vi "ReadConcTempPressureVer08.vi"() -> ()   [LabVIEW 2011]
uses:
  <vilib>/Utility/error.llb/DialogType.ctl
  <vilib>/Analysis/NI_AALBase.lvlib
panel:
  out "CPCconc":dbl=5620.0
  out "Smps Setting String":string
  in  "Allow SMPS scan":bool
  out "Saving in Progress":i32(slide) caption="Saving" scale=0.0..9.0
  out "Pressure (Hectopascal)":dbl=1011.5068458586213 format="%#.2f"
  out "Number Samples of Press.":dbl format="%.1f"
  out "Std error Press. to file (hpas)":dbl format="%.2f"
  out "Mean Press. to file (hpas)":dbl format="%.2f"
  in  "Std Press. error tolerance(%)":dbl=0.1 format="%.1f"
  out "Mean Pressure":dbl format="%.1f"
  out "Std Error Pressure (%)":dbl format="%.2f"
  out "Pressure Graph":cluster{"mean":dbl, dbl}(graph)={"mean"=1011.5068458586213, 1011.5068458586213} caption="Waveform Chart"
  out "Temperature(Celcius)":dbl=22.3189775953034 format="%#.2f"
  out "Number Samples of Temp":dbl format="%.1f"
  out "Std error Temp to file (deg)":dbl format="%.1f"
  out "Mean Temp to file (deg)":dbl format="%#.0f"
  in  "Std Temp error tolerance(%)":dbl=0.1 format="%.1f"
  out "Mean Temperature":dbl format="%.2f"
  out "Std Error Temp (%)":dbl format="%.2f"
  out "Temperature Graph":cluster{"mean":dbl, dbl}(graph)={"mean"=22.3189775953034, 22.3189775953034} caption="Waveform Chart"
  in  "CPC port":refnum<visa-resource-name>="COM4"
  out "Conc. (N/cm^3)":dbl=5620.0 format="%.1f"
  out "Number Samples of Conc.":dbl format="%.1f"
  out "Std error to file (N/cm^3)":dbl format="%.1f"
  out "Mean conc. to file (N/cm^3)":dbl format="%.2f"
  out "output array 2":dbl[](array[numeric])
  out "output 2":dbl
  out "output 1":dbl
  out "Std Error Concentration":dbl format="%.1f"
  in  "Std Conc. error tolerance(%)":dbl=0.1 format="%.1f"
  out "Std Concentration":dbl format="%.1f"
  out "Mean Conc.":dbl format="%.1f"
  out "Std Error Conc. (%)":dbl format="%.2f"
  out "output array":dbl[](array[numeric])=[5620.0, 5680.0, 5660.0, 5740.0, nan, 0.0, 0.0, 0.0, 0.0, 0.0, 0.0, 0.0, 0.0, 0.0, 0.0, 0.0, 0.0, 0.0, 0.0, 0.0, 0.0, 0.0, 0.0, 0.0, 0.0, 0.0, 0.0, 0.0, 0.0, 0.0]
  in  "Running Average Time(sec)":i32=30
  out "Particle Concentration from CPC":cluster{"mean":dbl, dbl}(graph)={"mean"=5620.0, 5620.0} caption="Waveform Chart"
  in  "OK":bool
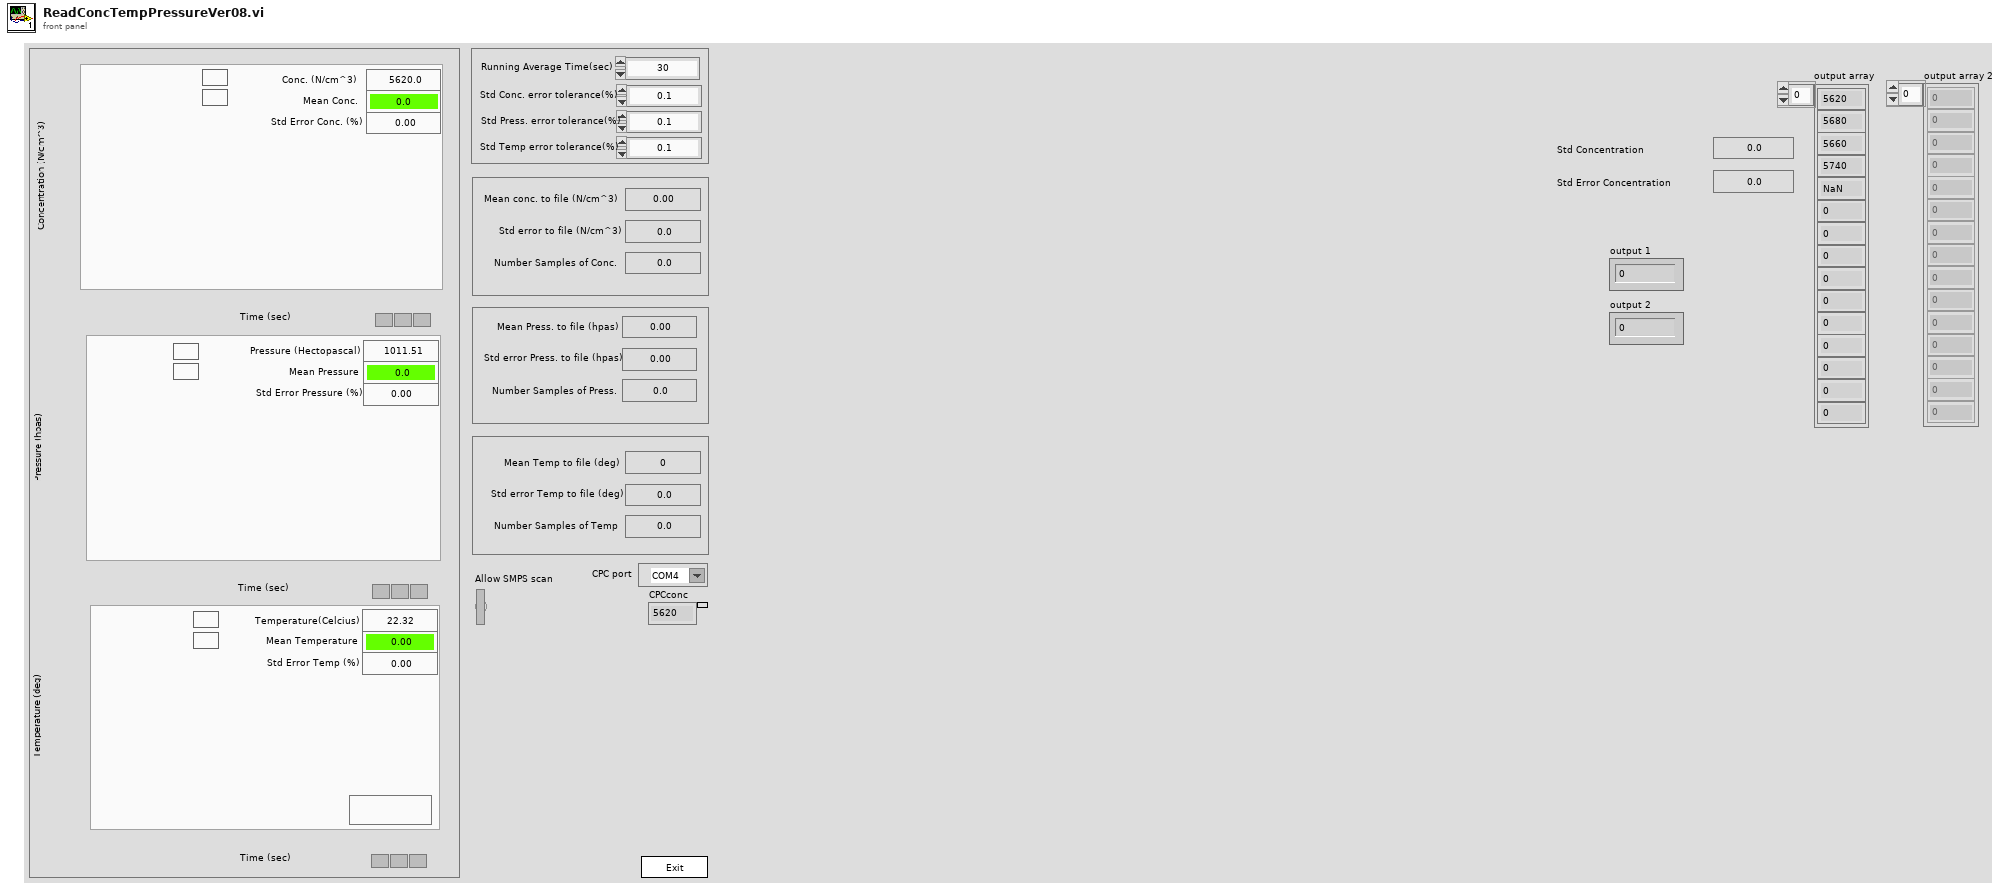
[diagram p1: front panel]
types:
  T1 = enum32{"invalid app kind", "Development System", "Run Time System", "Student Edition", "Embedded LabVIEW", "Evaluation", "Custom"}
  T2 = enum32{"Invalid", "Standard", "Closed", "Hidden", "Minimized", "Maximized"}
  T3 = cluster{"Core":cluster{"Current VI Reference":refnum<vi>, "Close Panel on Exit?":bool}, dbl[], "Running Average Time(sec)":i32, dbl[], "element":dbl, "dimension size":i32, "input file":path, "input file":path, "dup CPC port":refnum<visa-resource-name>, "CPC model":string, "input file":path, "input file":path, cluster{dbl[], dbl[], "element":dbl}, cluster{dbl[], dbl[], "element":dbl}}
  T4 = typedef "DialogType.ctl" = u16
  T5 = cluster{"Current VI Reference":refnum<vi>, "Close Panel on Exit?":bool}
  T6 = cluster{"concentration part/cm3":dbl, "concentration part/cm3":dbl}
  T7 = cluster{"concentration part/cm3":dbl, "mean":dbl}
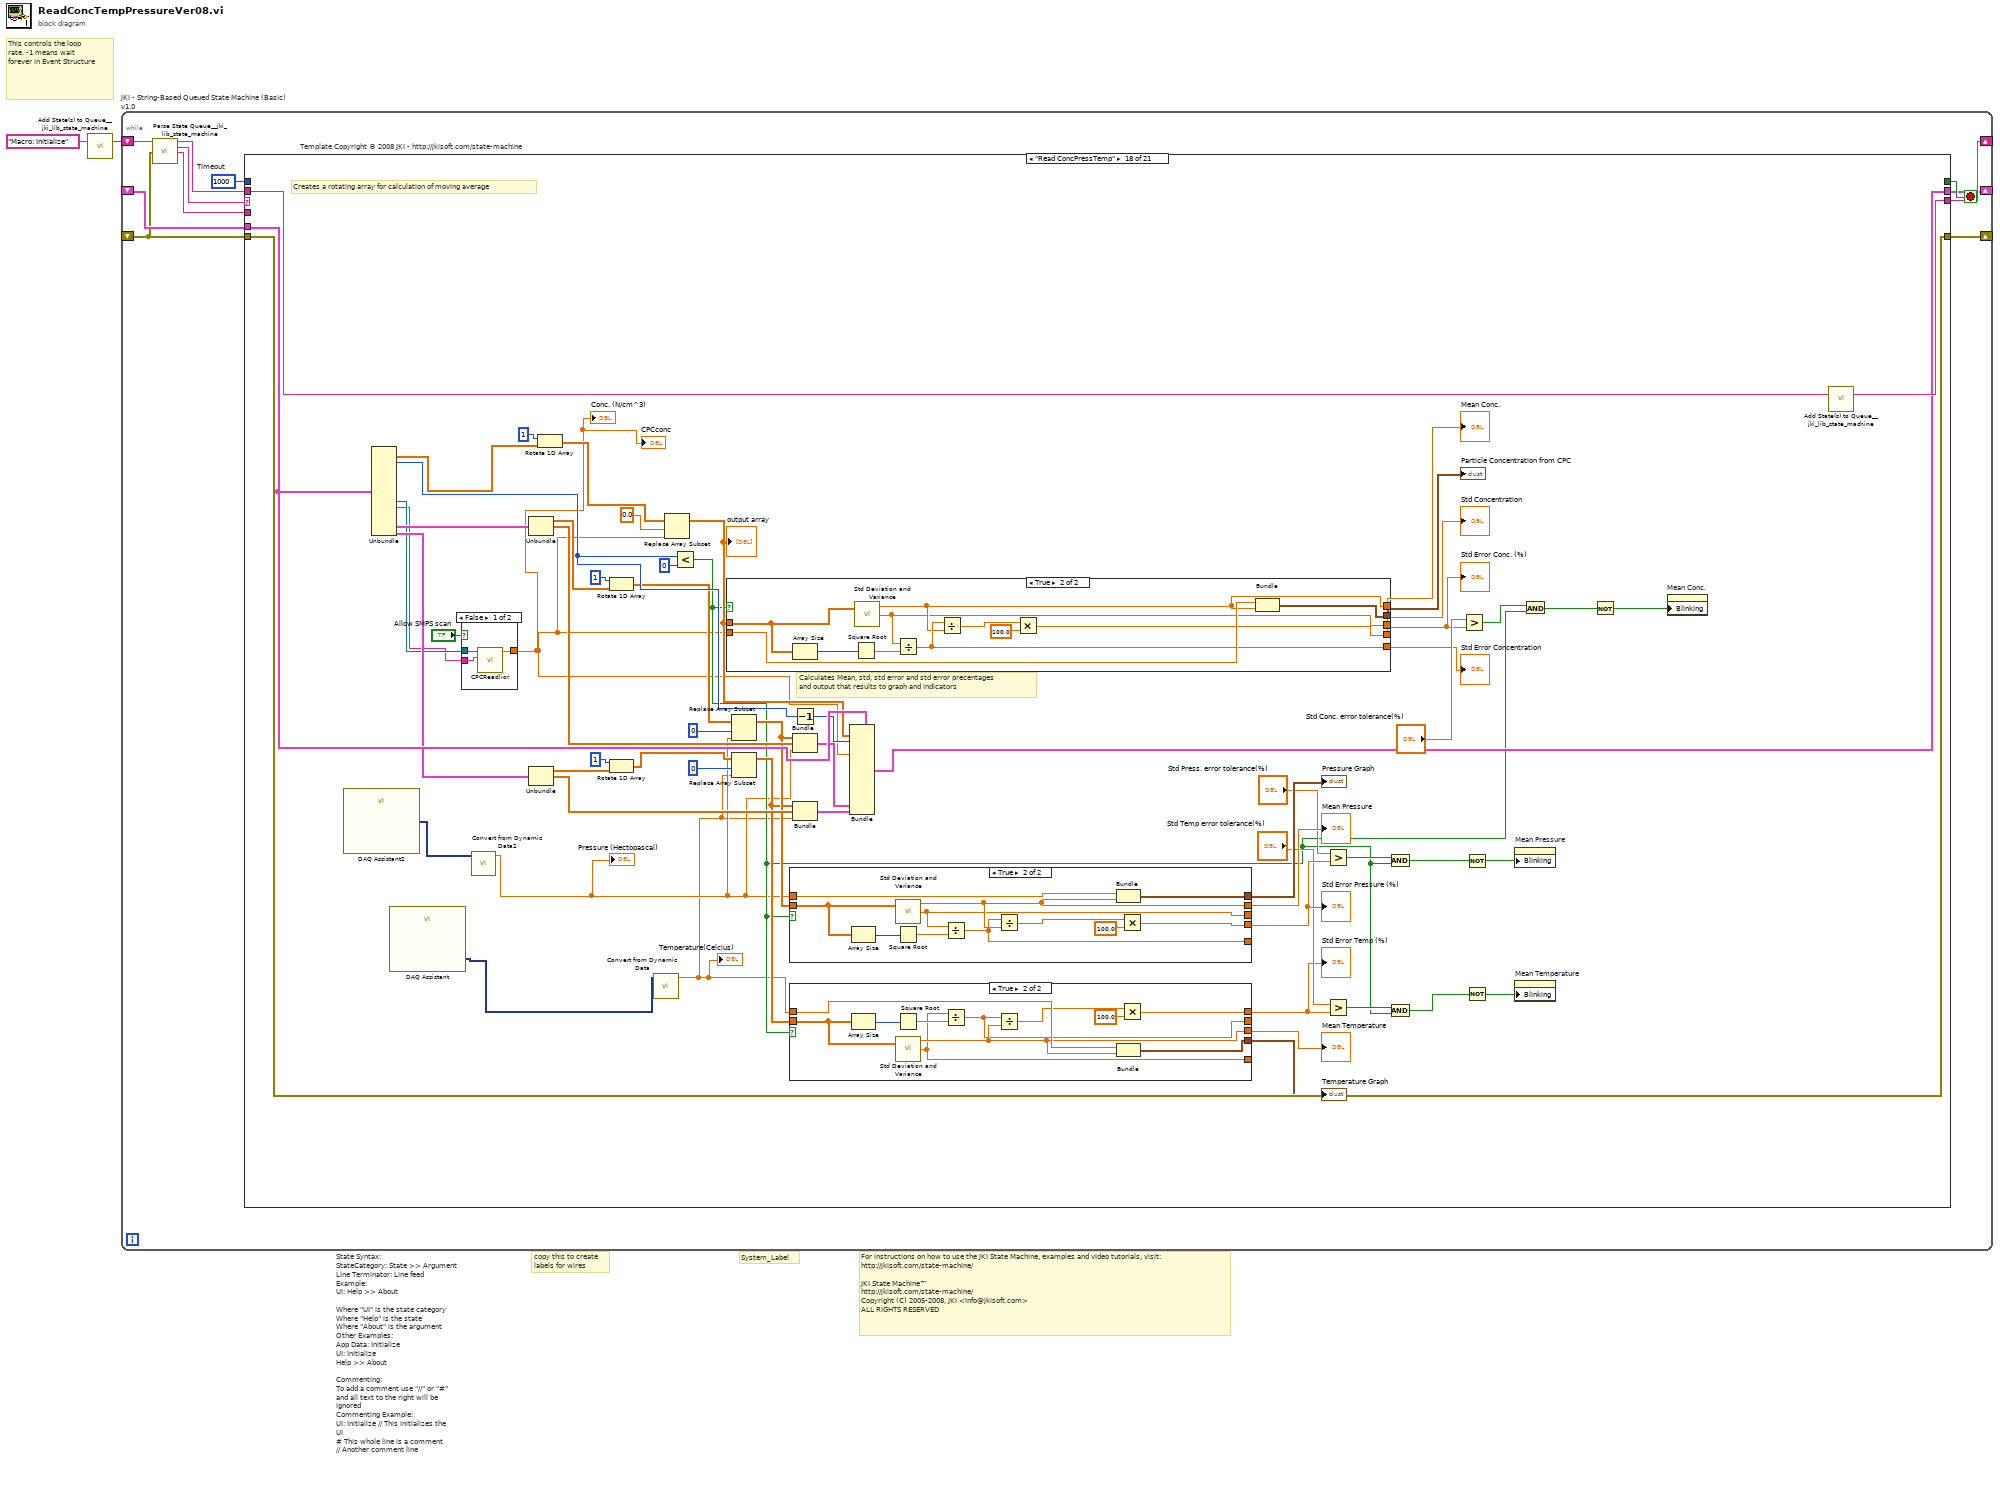
[diagram p0: block diagram]
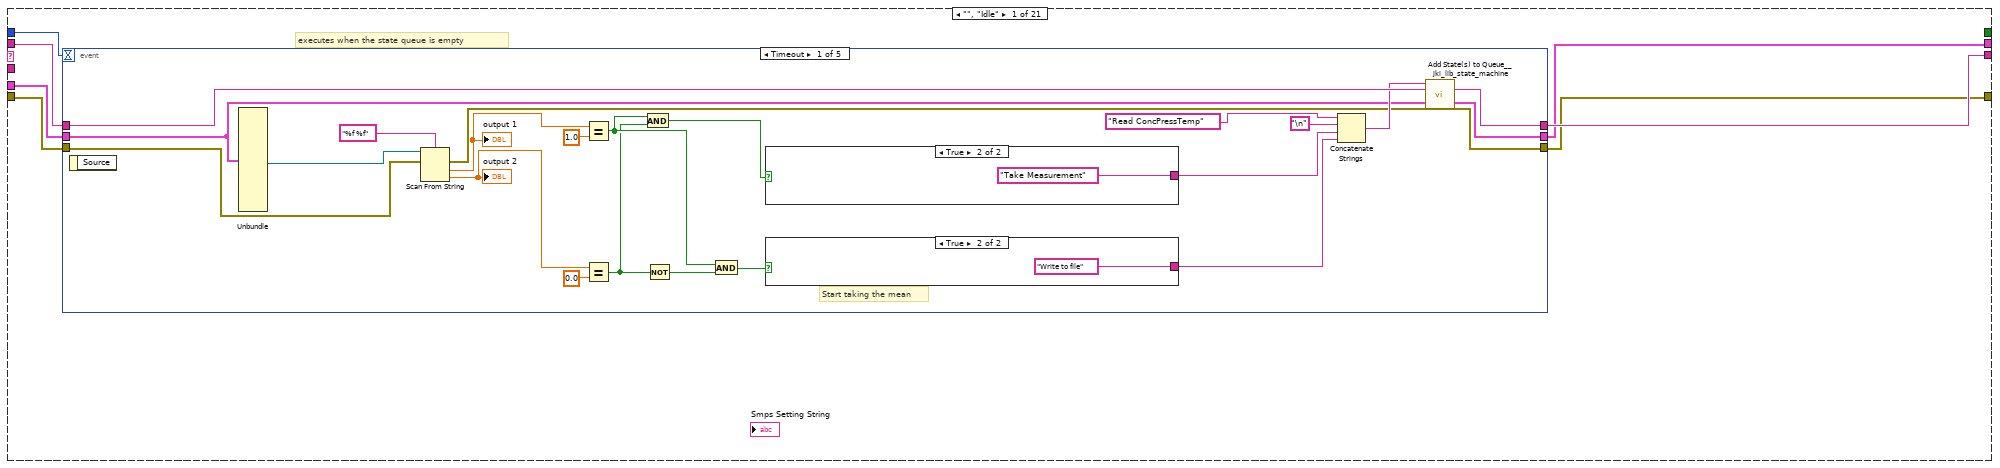
[diagram p2: hidden frame]
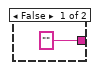
[diagram p3: hidden frame]
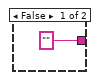
[diagram p4: hidden frame]
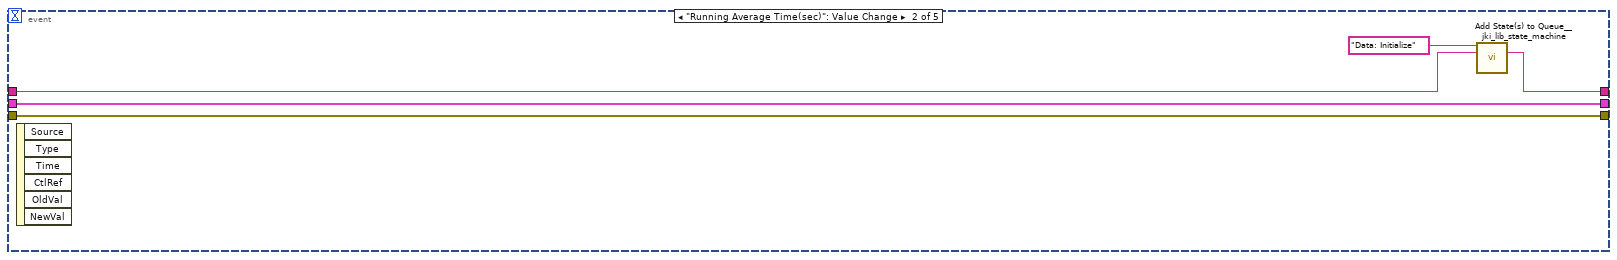
[diagram p5: hidden frame]
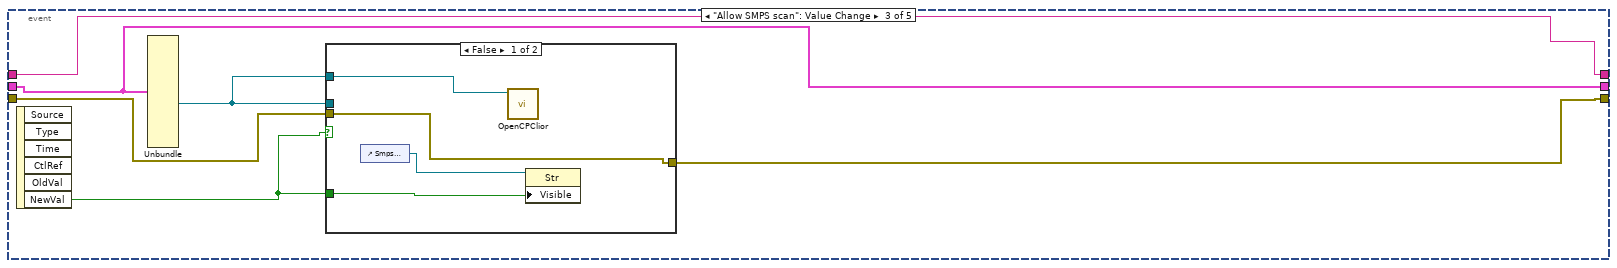
[diagram p6: hidden frame]
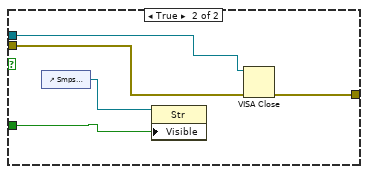
[diagram p7: hidden frame]
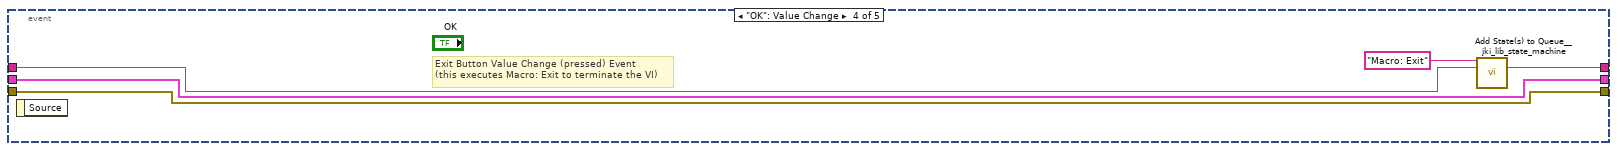
[diagram p8: hidden frame]
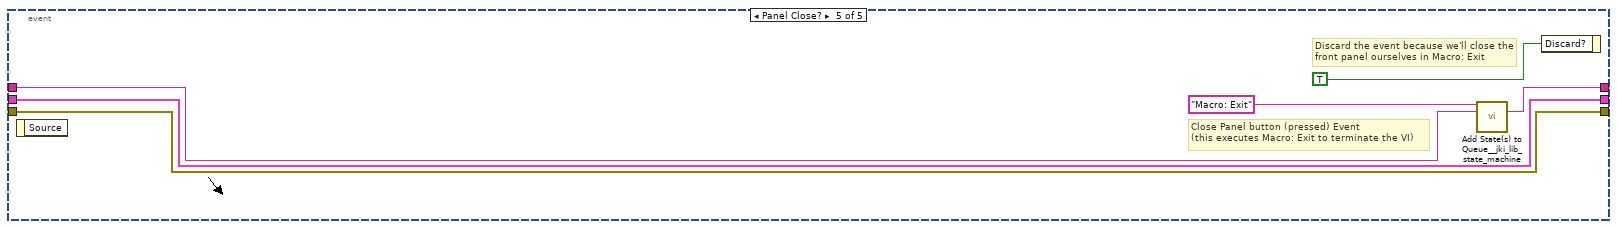
[diagram p9: hidden frame]
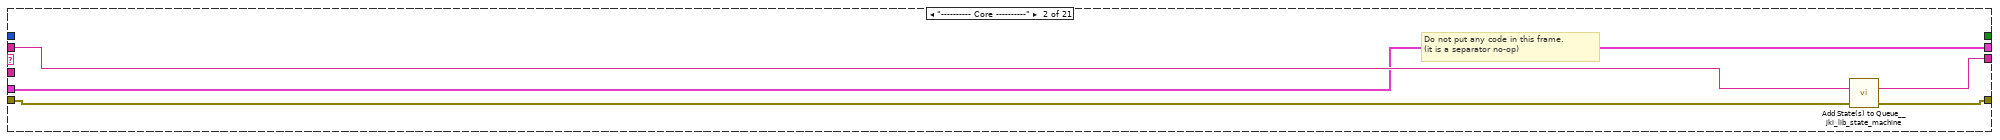
[diagram p10: hidden frame]
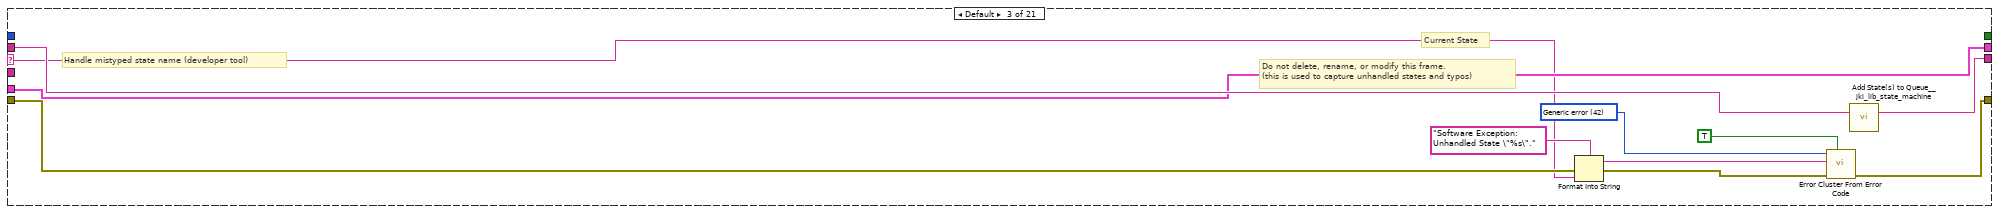
[diagram p11: hidden frame]
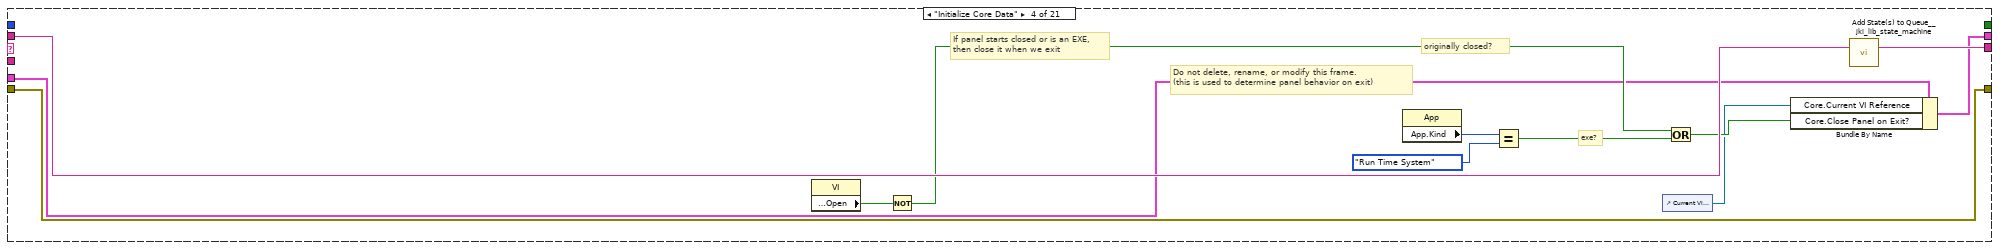
[diagram p12: hidden frame]
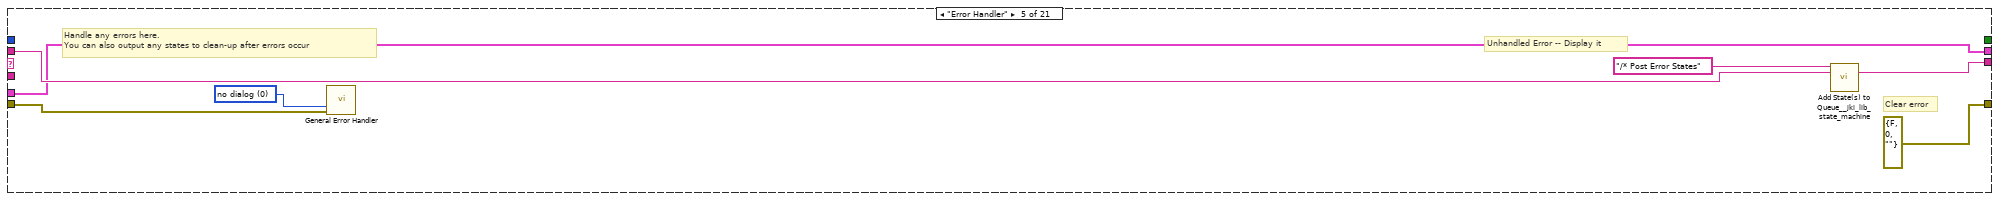
[diagram p13: hidden frame]
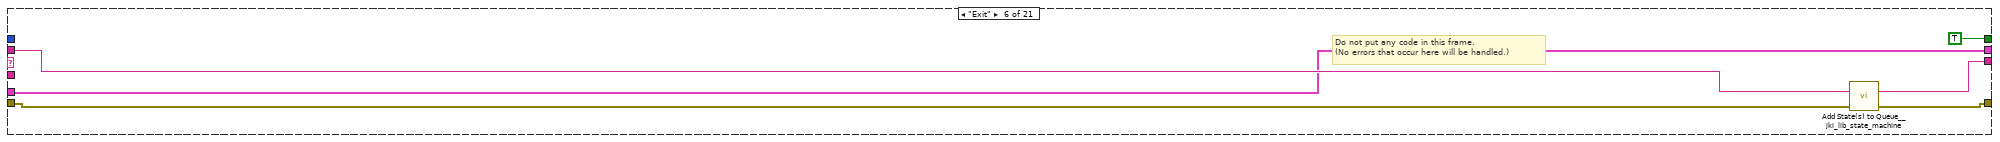
[diagram p14: hidden frame]
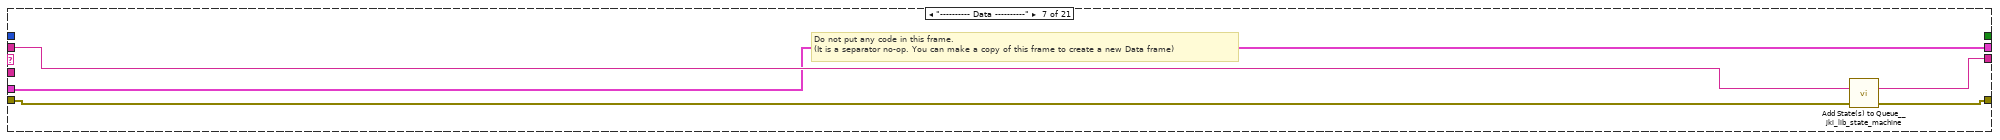
[diagram p15: hidden frame]
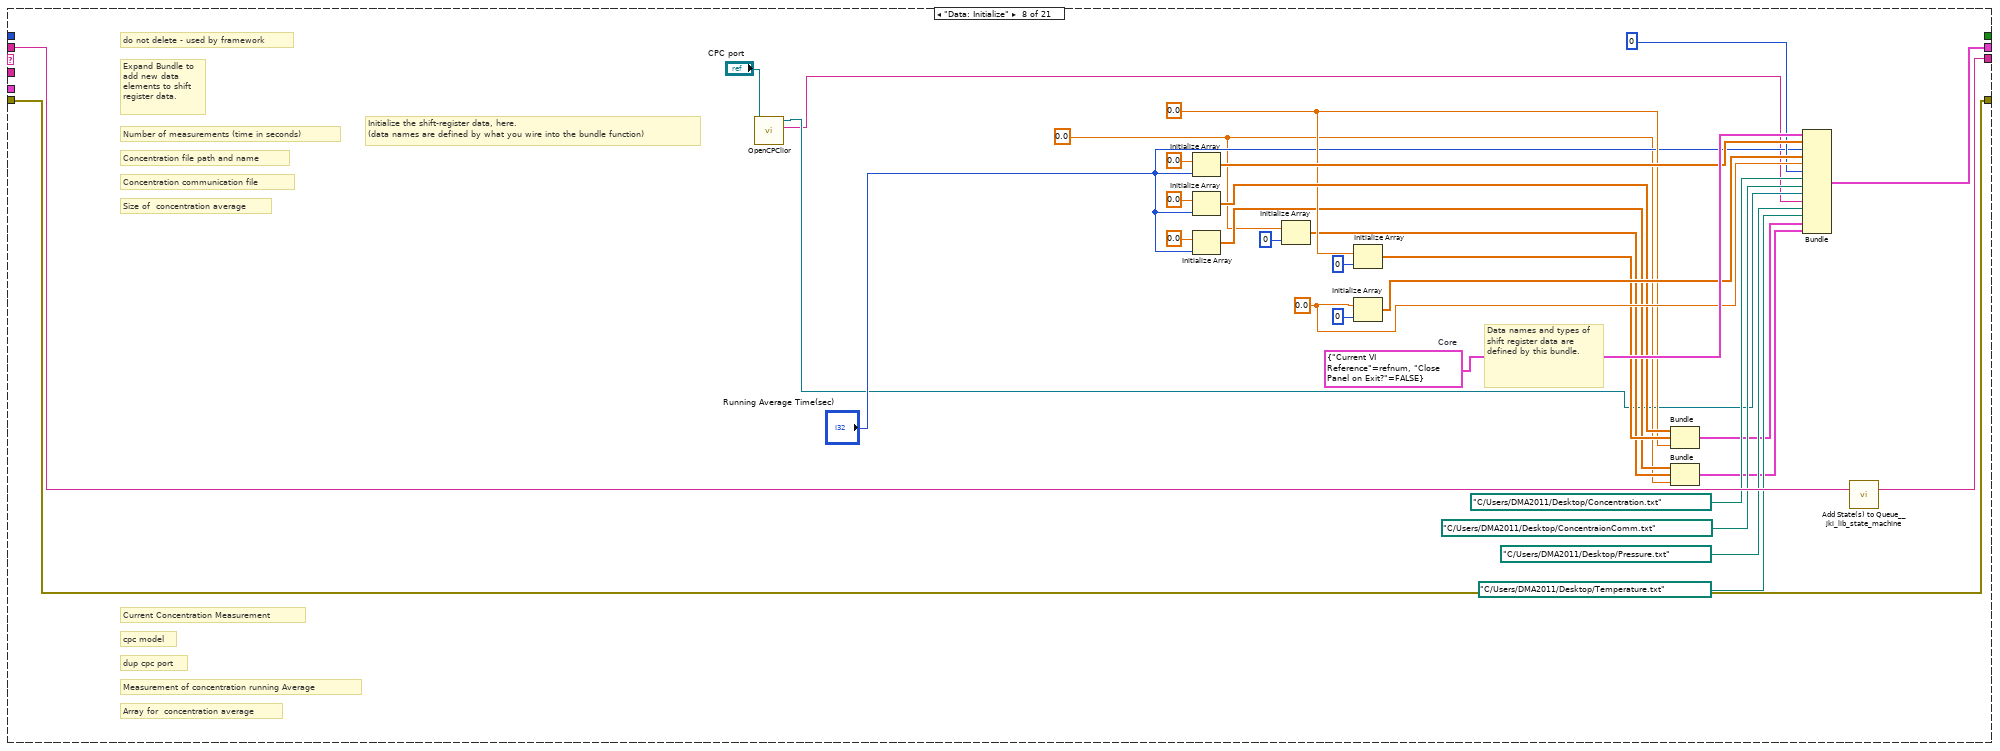
[diagram p16: hidden frame]
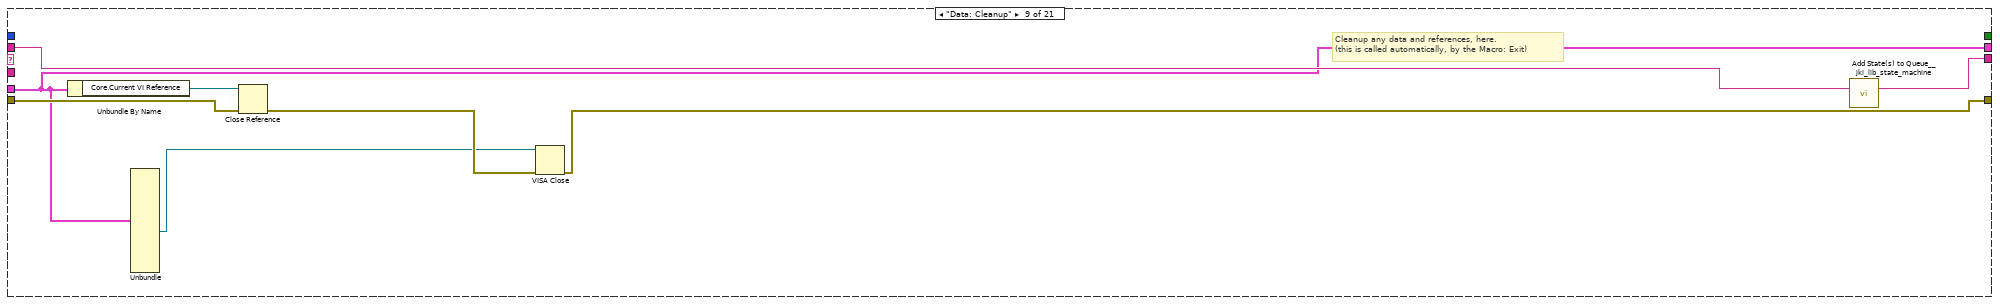
[diagram p17: hidden frame]
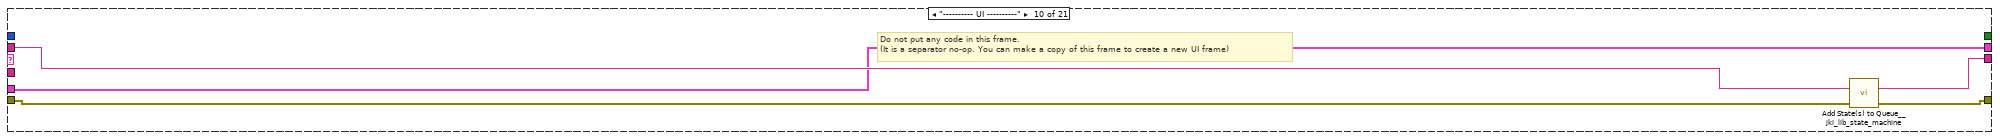
[diagram p18: hidden frame]
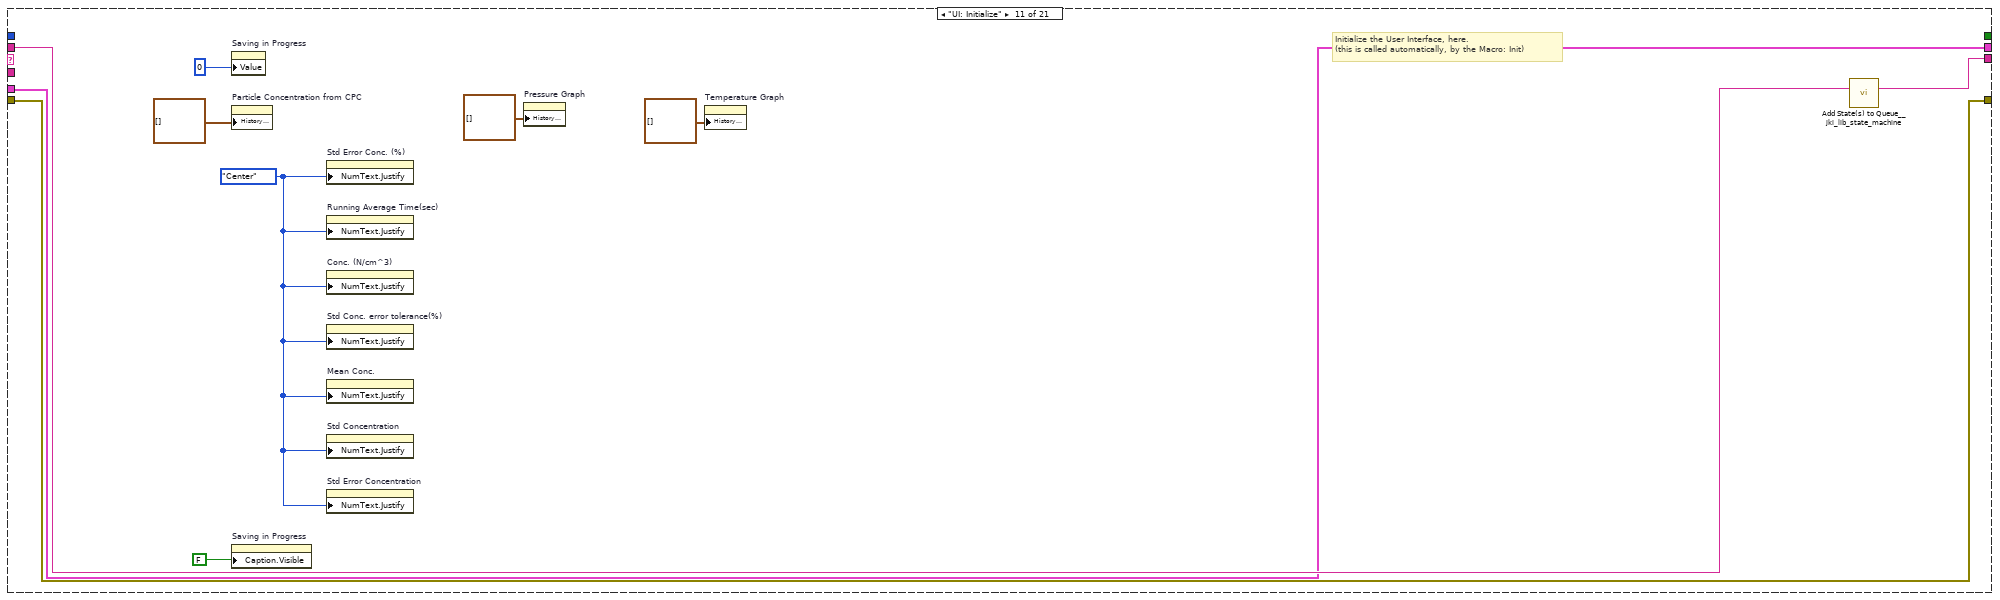
[diagram p19: hidden frame]
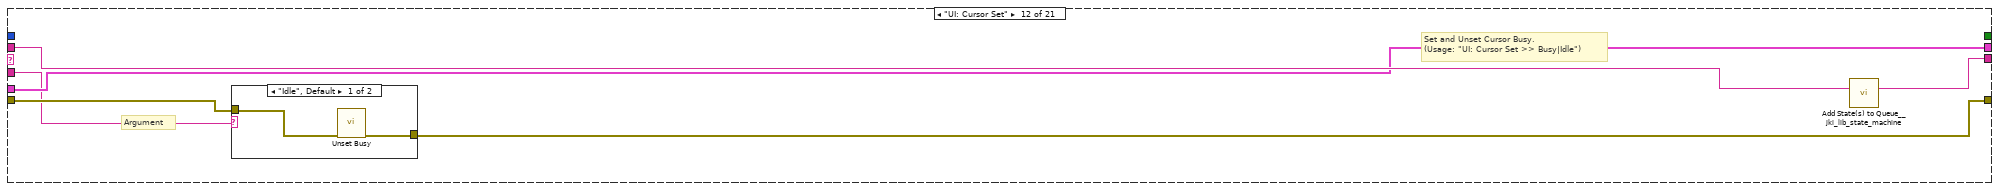
[diagram p20: hidden frame]
diagram:
  # "For instructions on how to use the JKI State Machine, examples and video tutorials, visit:\nhttp://jkisoft.com/state-machine/\n\nJKI State Machine™\nhttp://jkisoft.com/state-machine/\nCopyright (C) 2005-2008, JKI <info@jkisoft.com>\nALL RIGHTS RESERVED"
  # "State Syntax:\nStateCategory: State >> Argument\nLine Terminator: Line feed\nExample:\nUI: Help >> About\n\nWhere \"UI\" is the state category\nWhere \"Help\" is the state\nWhere \"About\" is the argument\nOther Examples:\nApp Data: Initialize\nUI: Initialize\nHelp >> About\n\nCommenting:\nTo add a comment use \"//\" or \"#\" and all text to the right will be ignored\nCommenting Example:\nUI: Initialize // This initializes the UI\n# This whole line is a comment\n// Another comment line"
  # "copy this to create labels for wires"
  # "This controls the loop rate. -1 means wait forever in Event Structure"
  # "System_Label"
  n1 = call <vilib>:"Add State(s) to Queue__jki_lib_state_machine.vi"("State(s) in (\"\")"="Macro: Initialize") -> ("States Out"=w2:string)  [unwired: 14 in]
  n2 = while "JKI - String-Based Queued State Machine (Basic) v1.0" {
    shift-right: [w6] -> _
    shift-left: _ -> [w5]
    shift-right: [w9] -> _
    shift-left: _ -> [w3]
    shift-right: [w8] -> _
    shift-left: w2 -> [w10]
    stop <- w7 stop-if-true
    w4 = 1000  # Timeout
    # "Template Copyright © 2008 JKI - http://jkisoft.com/state-machine"
    n3 = call <vilib>:"Parse State Queue__jki_lib_state_machine.vi"("State Queue"=w10, "Error In (no error)"=w3) -> ("Remaining States"=w12:string, "Current State"=w13:string, "Arguments"=w11:string)  [unwired: 11 in]
    n4 = case shown="\"Read ConcPressTemp\"" w13 {
      selector: w13 -> [_ _ w81 _ _ _ _ _ _ _ _ _ _ _ _ _ _ _ _ _ _]
      tunnel: w12 -> [w20 w80 w85 w103 w110 w115 w119 w150 w158 w162 w172 w178 w189 w215 w220 w230 w234 w295 w345 w375 w435]
      tunnel: w11 -> [_ _ _ _ _ _ _ _ _ _ _ w173 w183 _ _ _ _ _ _ _ _]
      tunnel: w5 -> [w18 w77 w83 w94 w107 w113 w116 _ w152 w159 w170 w176 w185 w212 w217 w227 w231 w291 w342 w369 w424]
      tunnel: [w17 w78 w87 w100 errorcluster {"status"=FALSE, "code"=0, "source"=""} ("error out") w112 w117 w147 w153 w160 w169 w174 w186 w213 w218 w228 w232 w293 w343 w373 w398] -> w9
      tunnel: w3 -> [w16 w78 w86 w100 w106 w112 w117 w147 w155 w160 w169 w175 w187 w213 w218 w228 w232 w293 w343 w373 w413]
      tunnel: [w19 w79 w84 w102 w109 w114 w118 w149 w157 w161 w171 w177 w188 w214 w219 w229 w233 w294 w344 w374 w434] -> w8
      tunnel: [_ _ _ _ _ TRUE _ _ _ _ _ _ _ _ _ _ _ _ _ _ _] -> w7
      tunnel: [w15 w77 w83 w101 w107 w113 w116 w148 w152 w159 w170 w176 w185 w212 w217 w227 w231 w292 w342 w368 w423] -> w6
      tunnel: w4 -> [w14 _ _ _ _ _ _ _ _ _ _ _ _ _ _ _ _ _ _ _ _]
      frame "", "Idle" {
        # "executes when the state queue is empty"
        n5 = event shown="[0] Timeout" {
          selector: _ -> [_ _ _ _ _]
          dyn-events: _ -> [_ _ _ _ _]
          timeout: w14 -> [_ _ _ _ _]
          tunnel: w20 -> [w41 w50 w53 w70 w76]
          tunnel: [w40 w49 w53 w69 w75] -> w19
          tunnel: w18 -> [w24 w47 w52 w67 w73]
          tunnel: [w21 w48 w55 w68 w74] -> w17
          tunnel: w16 -> [w22 w48 w56 w68 w74]
          tunnel: [w24 w47 w52 w67 w73] -> w15
          event Timeout {
            # "Start taking the mean"
            n6 = event-data() -> ()  [unwired: 1 in, 1 out]
            n7 = Unbundle(w24) -> ("input file"=w23:path)  [unwired: 13 out]
            n8 = Scan From String("%f %f" ("format string"), w23, w22) -> (w21:errorcluster, output 1=w38:dbl, output 2=w35:dbl)  [unwired: 2 in, 1 out]
            "output 1" <- w38
            "output 2" <- w35
            n9 = Equal?(x=w38, y=1.0) -> (x = y?=w29:bool)
            n10 = Equal?(x=w35, y=0.0) -> (x = y?=w27:bool)
            n11 = And(x=w29, y=w27) -> (x .and. y?=w34:bool)
            n12 = Not(x=w27) -> (.not. x?=w28:bool)
            n13 = And(x=w29, y=w28) -> (x .and. y?=w26:bool)
            n14 = case shown="True" w34 {
              tunnel: ["" ("State(s) in Front (\"\")") "Take Measurement" ("State(s) in Front (\"\")")] -> w30
              frame False {
              }
              frame True {
              }
            }
            n15 = case shown="True" w26 {
              tunnel: ["" ("State(s) in Front (\"\")") "Write to file" ("State(s) in Front (\"\")")] -> w25
              frame False {
              }
              frame True {
              }
            }
            n16 = Concatenate Strings("Read ConcPressTemp" ("State(s) in Front (\"\")"), "\n", w30, w25) -> (w33:string)
            n17 = call <vilib>:"Add State(s) to Queue__jki_lib_state_machine.vi"("State(s) in Front (\"\")"=w33, "State(s) in (\"\")"=w41) -> ("States Out"=w40:string)  [unwired: 13 in]
          }
          event "Running Average Time(sec)": Value Change {
            n18 = event-data() -> ()  [unwired: 1 in, 6 out]
            n19 = call <vilib>:"Add State(s) to Queue__jki_lib_state_machine.vi"("State(s) in Front (\"\")"="Data: Initialize" ("State(s) in Front (\"\")"), "State(s) in (\"\")"=w50) -> ("States Out"=w49:string)  [unwired: 13 in]
          }
          event "Allow SMPS scan": Value Change {
            n20 = event-data() -> ("NewVal"=w51:bool)  [unwired: 1 in, 5 out]
            n21 = Unbundle(w52) -> ("dup CPC port"=w54:refnum<visa-resource-name>)  [unwired: 13 out]
            n22 = case shown="False" w51 {
              tunnel: w54 -> [_ w65]
              tunnel: w56 -> [w59 w64]
              tunnel: [w59 w63] -> w55
              tunnel: w54 -> [w60 _]
              tunnel: w51 -> [w57 w61]
              frame False {
                n23 = control-ref of="Smps Setting String"() -> (w58:refnum<vi>)
                n24 = call "OpenCPClior.vi"("CPC port"=w60) -> ()  [unwired: 8 in, 3 out]
                n25 = property on="Property Node" class="Str"(reference=w58, "Visible"=w57) -> ()  [unwired: 1 in, 2 out]
              }
              frame True {
                n26 = control-ref of="Smps Setting String"() -> (w62:refnum<vi>)
                n27 = property on="Property Node" class="Str"(reference=w62, "Visible"=w61) -> ()  [unwired: 1 in, 2 out]
                n28 = VISA Close(VISA resource name=w65, error in (no error)=w64) -> (error out=w63:errorcluster)
              }
            }
          }
          event "OK": Value Change {
            # "Exit Button Value Change (pressed) Event\n(this executes Macro: Exit to terminate the VI)"
            n29 = event-data() -> ()  [unwired: 1 in, 1 out]
            n30 = call <vilib>:"Add State(s) to Queue__jki_lib_state_machine.vi"("State(s) in Front (\"\")"="Macro: Exit", "State(s) in (\"\")"=w70) -> ("States Out"=w69:string)  [unwired: 13 in]
          }
          event Panel Close? {
            # "Discard the event because we'll close the front panel ourselves in Macro: Exit"
            # "Close Panel button (pressed) Event\n(this executes Macro: Exit to terminate the VI)"
            n31 = event-data() -> ()  [unwired: 1 in, 1 out]
            n32 = call <vilib>:"Add State(s) to Queue__jki_lib_state_machine.vi"("State(s) in Front (\"\")"="Macro: Exit", "State(s) in (\"\")"=w76) -> ("States Out"=w75:string)  [unwired: 13 in]
            n33 = event-data("Discard?"=TRUE) -> ()  [unwired: 1 in, 1 out]
          }
        }
      }
      frame "---------- Core ----------" {
        # "Do not put any code in this frame.\n(it is a separator no-op)"
        n34 = call <vilib>:"Add State(s) to Queue__jki_lib_state_machine.vi"("State(s) in (\"\")"=w80) -> ("States Out"=w79:string)  [unwired: 14 in]
      }
      frame Default {
        w90 = 42 items=["No error", "Argument error", "Memory is full", "Out of zone", "End of file", "File already open", "Generic file I/O error", "File not found", "File permission error", "Disk is full", "Duplicate path", "Too many files open", "System feature not enabled", "Resource file not found", "Cannot add resource", "Resource not found", "Image not found", "Image memory error", "Pen does not exist", "Config type invalid", "Config token not found", "Config parse error", "Config memory error", "Bad external code format", "Bad external code offset", "External code not present", "Null window", "Destroy window error", "Null menu", "Print aborted", "Bad print record", "Print driver error", "Windows error during printing", "Memory error during printing", "Print dialog error", "Generic print error", "Invalid device refnum", "Device not found", "Device parameter error", "Device unit error", "Cannot open device", "Device call aborted", "Generic error", "Cancelled by user", "Object ID too low", "Object ID too high", "Object not in heap", "Unknown heap", "Unknown object (invalid DefProc)", "Unknown object (DefProc not in table)", "Message out of range", "Invalid (null) method", "Unknown message", "Manager call not supported", "Bad address", "Network operation in progress", "Network operation timed out", "Connection is busy", "Network attribute not supported", "Network error", "Address in use", "System out of memory", "Connection aborted", "Connection refused", "Not connected", "Already connected", "Connection closed", "Initialization error (interapplication manager)", "Bad occurrence", "Wait on unbound occurrence handler", "Occurrence queue overflow", "Datalog type conflict", "Unused", "Unrecognized type (interapplication manager)", "Memory corrupt", "Failed to make temporary DLL", "Old CIN version", "Drag socket not found", "Failed to load drop-object", "Failed to register OLE object", "Failed to release OLE object", "Format specifier type mismatch", "Unknown format specifier", "Too few format specifiers", "Too many format specifiers", "Scan failed", "Newer CIN version", "Error converting to variant", "Runtime menu error", "Password tampered", "Variant attribute not found", "Incompatible variant data type", "Event data is not available", "Event Store is not present", "Occurrence is not found", "Event Queue is not created", "Event info is not available", "Refnum passed is NULL", "Error retrieving Class GUID", "Error retrieving CoClass GUID", "Error retrieving TypeLib GUID.", "Bad built application magic bytes.", "Specific driver is different from the specific driver associated with the Logical Name.", "There is no session opened to the class driver.", "Max Error", "MAX - Error with config objects", "MAX - Error loading configuration", "MAX - Group not supported"]
        # "Current State"
        # "Do not delete, rename, or modify this frame.\n(this is used to capture unhandled states and typos)"
        # "Handle mistyped state name (developer tool)"
        n35 = Format Into String(format string="Software Exception: Unhandled State \"%s\"." ("message"), error in=w86, w81) -> (resulting string=w89:string, error out=w88:errorcluster)  [unwired: 1 in]
        n36 = call <vilib>:"Error Cluster From Error Code.vi"("show call chain? (False)"=TRUE, "error in (no error)"=w88, "error message (\"\")"=w89, "error code (0)"=w90) -> ("error out"=w87:errorcluster)  [unwired: 5 in]
        n37 = call <vilib>:"Add State(s) to Queue__jki_lib_state_machine.vi"("State(s) in (\"\")"=w85) -> ("States Out"=w84:string)  [unwired: 14 in]
      }
      frame "Initialize Core Data" {
        # "Do not delete, rename, or modify this frame.\n(this is used to determine panel behavior on exit)"
        # "originally closed?"
        # "exe?"
        # "If panel starts closed or is an EXE, then close it when we exit"
        n38 = property class="VI"() -> ("Front Panel.Open"=w99:bool)  [unwired: 2 in, 2 out]
        n39 = Not(x=w99) -> (.not. x?=w96:bool)
        n40 = property class="App"() -> ("App.Kind"=w98:T1)  [unwired: 2 in, 2 out]
        n41 = Equal?(x=w98, y=T1."Run Time System" ("Application:Kind")) -> (x = y?=w95:bool)
        n42 = control-ref of="Current VI Reference"() -> (w92:refnum<vi>)
        n43 = Or(x=w96, y=w95) -> (x .or. y?=w93:bool)
        n44 = Bundle By Name(cluster=w94, "Core.Current VI Reference"=w92, "Core.Close Panel on Exit?"=w93) -> (w101:T3)
        n45 = call <vilib>:"Add State(s) to Queue__jki_lib_state_machine.vi"("State(s) in (\"\")"=w103) -> ("States Out"=w102:string)  [unwired: 14 in]
      }
      frame "Error Handler" {
        w104 = T4 0 items=["no dialog", "OK message", "continue or stop message", "OK message + warnings", "continue/stop + warnings"] ("type of dialog (OK msg:1)")
        # "Unhandled Error -- Display it"
        # "Handle any errors here.\nYou can also output any states to clean-up after errors occur"
        # "Clear error"
        n46 = call <vilib>:"General Error Handler.vi"("type of dialog (OK msg:1)"=w104, "error in (no error)"=w106) -> ()  [unwired: 9 in, 5 out]
        n47 = call <vilib>:"Add State(s) to Queue__jki_lib_state_machine.vi"("State(s) in Front (\"\")"="/* Post Error States", "State(s) in (\"\")"=w110) -> ("States Out"=w109:string)  [unwired: 13 in]
      }
      frame "Exit" {
        # "Do not put any code in this frame.\n(No errors that occur here will be handled.)"
        n48 = call <vilib>:"Add State(s) to Queue__jki_lib_state_machine.vi"("State(s) in (\"\")"=w115) -> ("States Out"=w114:string)  [unwired: 14 in]
      }
      frame "---------- Data ----------" {
        # "Do not put any code in this frame.\n(It is a separator no-op. You can make a copy of this frame to create a new Data frame)"
        n49 = call <vilib>:"Add State(s) to Queue__jki_lib_state_machine.vi"("State(s) in (\"\")"=w119) -> ("States Out"=w118:string)  [unwired: 14 in]
      }
      frame "Data: Initialize" {
        w123 = 0.0 ("element")
        w130 = 0.0 ("element")
        w141 = 0.0 ("element")
        w146 = T5 {"Current VI Reference"=refnum, "Close Panel on Exit?"=FALSE}  # Core
        # "cpc model"
        # "dup cpc port"
        # "Concentration communication file"
        # "Concentration file path and name"
        # "Number of measurements (time in seconds)"
        # "Current Concentration Measurement"
        # "Size of  concentration average"
        # "Array for  concentration average"
        # "Measurement of concentration running Average"
        # "do not delete - used by framework"
        # "Expand Bundle to add new data elements to shift register data."
        # "Data names and types of shift register data are defined by this bundle."
        # "Initialize the shift-register data, here.\n(data names are defined by what you wire into the bundle function)"
        n50 = call "OpenCPClior.vi"("CPC port"="CPC port") -> ("CPC model"=w120:string, "dup CPC port"=w121:refnum<visa-resource-name>)  [unwired: 8 in, 1 out]
        n51 = Initialize Array(0.0 ("element"), "Running Average Time(sec)") -> (w144:dbl[])
        n52 = Initialize Array(0.0 ("element"), "Running Average Time(sec)") -> (w134:dbl[])
        n53 = Initialize Array(0.0 ("element"), "Running Average Time(sec)") -> (w127:dbl[])
        n54 = Initialize Array(w123, 0 ("dimension size")) -> (w124:dbl[])
        n55 = Initialize Array(w130, 0 ("dimension size")) -> (w131:dbl[])
        n56 = Initialize Array(w141, 0 ("dimension size")) -> (w142:dbl[])
        n57 = Bundle(w134, w131, "element"=w130) -> (w133:cluster{dbl[], dbl[], "element":dbl})  [unwired: 1 in]
        n58 = Bundle(w127, w124, "element"=w123) -> (w129:cluster{dbl[], dbl[], "element":dbl})  [unwired: 1 in]
        n59 = Bundle("Core"=w146, w144, "Running Average Time(sec)"="Running Average Time(sec)", w142, "element"=w141, "dimension size"=0, "input file"=path "C:/Users/DMA2011/Desktop/Concentration.txt", "input file"=path "C:/Users/DMA2011/Desktop/ConcentraionComm.txt", "dup CPC port"=w121, "CPC model"=w120, "input file"=path "C:/Users/DMA2011/Desktop/Pressure.txt", "input file"=path "C:/Users/DMA2011/Desktop/Temperature.txt", w133, w129) -> (w148:T3)  [unwired: 1 in]
        n60 = call <vilib>:"Add State(s) to Queue__jki_lib_state_machine.vi"("State(s) in (\"\")"=w150) -> ("States Out"=w149:string)  [unwired: 14 in]
      }
      frame "Data: Cleanup" {
        # "Cleanup any data and references, here.\n(this is called automatically, by the Macro: Exit)"
        n61 = Unbundle By Name(w152) -> ("Core.Current VI Reference"=w156:refnum<vi>)
        n62 = Unbundle(w152) -> ("dup CPC port"=w151:refnum<visa-resource-name>)  [unwired: 13 out]
        n63 = Close Reference(reference=w156, error in (no error)=w155) -> (error out=w154:errorcluster)
        n64 = VISA Close(VISA resource name=w151, error in (no error)=w154) -> (error out=w153:errorcluster)
        n65 = call <vilib>:"Add State(s) to Queue__jki_lib_state_machine.vi"("State(s) in (\"\")"=w158) -> ("States Out"=w157:string)  [unwired: 14 in]
      }
      frame "---------- UI ----------" {
        # "Do not put any code in this frame.\n(It is a separator no-op. You can make a copy of this frame to create a new UI frame)"
        n66 = call <vilib>:"Add State(s) to Queue__jki_lib_state_machine.vi"("State(s) in (\"\")"=w162) -> ("States Out"=w161:string)  [unwired: 14 in]
      }
      frame "UI: Initialize" {
        w166 = enum16{"Left", "Center", "Right"}."Center" ("Numeric Text.Justification")
        # "Initialize the User Interface, here.\n(this is called automatically, by the Macro: Init)"
        n67 = property on="Saving in Progress" class="Slide (strict)"("Value"=0 ("Saving in Progress")) -> ()  [unwired: 2 in, 2 out]
        n68 = property on="Particle Concentration from CPC" class="WFChart (strict)"("History Data"=cluster{"mean":dbl, dbl}[] []) -> ()  [unwired: 2 in, 2 out]
        n69 = property on="Saving in Progress" class="Slide (strict)"("Caption.Visible"=FALSE) -> ()  [unwired: 2 in, 2 out]
        n70 = property on="Std Error Conc. (%)" class="DigNum (strict)"("NumText.Justify"=w166) -> ()  [unwired: 2 in, 2 out]
        n71 = property on="Running Average Time(sec)" class="DigNum (strict)"("NumText.Justify"=w166) -> ()  [unwired: 2 in, 2 out]
        n72 = property on="Conc. (N/cm^3)" class="DigNum (strict)"("NumText.Justify"=w166) -> ()  [unwired: 2 in, 2 out]
        n73 = property on="Std Conc. error tolerance(%)" class="DigNum (strict)"("NumText.Justify"=w166) -> ()  [unwired: 2 in, 2 out]
        n74 = property on="Mean Conc." class="DigNum (strict)"("NumText.Justify"=w166) -> ()  [unwired: 2 in, 2 out]
        n75 = property on="Std Concentration" class="DigNum (strict)"("NumText.Justify"=w166) -> ()  [unwired: 2 in, 2 out]
        n76 = property on="Std Error Concentration" class="DigNum (strict)"("NumText.Justify"=w166) -> ()  [unwired: 2 in, 2 out]
        n77 = property on="Pressure Graph" class="WFChart (strict)"("History Data"=cluster{"mean":dbl, dbl}[] []) -> ()  [unwired: 2 in, 2 out]
        n78 = property on="Temperature Graph" class="WFChart (strict)"("History Data"=cluster{"mean":dbl, dbl}[] []) -> ()  [unwired: 2 in, 2 out]
        n79 = call <vilib>:"Add State(s) to Queue__jki_lib_state_machine.vi"("State(s) in (\"\")"=w172) -> ("States Out"=w171:string)  [unwired: 14 in]
      }
      frame "UI: Cursor Set" {
        # "Argument"
        # "Set and Unset Cursor Busy.\n(Usage: \"UI: Cursor Set >> Busy|Idle\")"
        n80 = case shown="\"Idle\", Default" w173 {
          tunnel: w175 -> [w180 w182]
          tunnel: [w179 w181] -> w174
          frame "Idle", Default {
            n81 = call <vilib>:"Unset Busy.vi"("error in (no error)"=w180) -> ("error out"=w179:errorcluster)  [unwired: 10 in]
          }
          frame "Busy" {
            n82 = call <vilib>:"Set Busy.vi"("error in (no error)"=w182) -> ("error out"=w181:errorcluster)  [unwired: 9 in, 1 out]
          }
        }
        n83 = call <vilib>:"Add State(s) to Queue__jki_lib_state_machine.vi"("State(s) in (\"\")"=w178) -> ("States Out"=w177:string)  [unwired: 14 in]
      }
      frame "UI: Front Panel State" {
        # "Argument"
        # "Set Front Panel Open or Closed\n(Usage: \"UI: Front Panel State >> Open|Close\")"
        n84 = Unbundle By Name(w185) -> ("Core.Current VI Reference"=w184:refnum<vi>)
        n85 = case shown="\"Open\", Default" w183 {
          tunnel: w187 -> [w193 w206]
          tunnel: [w195 w207] -> w186
          tunnel: w184 -> [w194 w204]
          frame "Open", Default {
            n86 = property class="VI"(reference=w194, error in=w193) -> (reference out=w191:refnum<vi>, error out=w192:errorcluster, "Front Panel.Open"=w190:bool)
            n87 = case shown="False" w190 {
              tunnel: [w198 w201] -> w195
              tunnel: w192 -> [w197 w201]
              tunnel: w191 -> [w196 _]
              frame False {
                n88 = invoke class="VI" method="FP.Open"(reference=w196, error in=w197, "Activate"=TRUE, "State"=T2."Standard") -> (error out=w198:errorcluster)  [unwired: 1 in, 4 out]
              }
              frame True {
              }
            }
          }
          frame "Close" {
            n89 = property class="VI"(reference=w204, error in=w206) -> (reference out=w203:refnum<vi>, error out=w205:errorcluster, "Front Panel.Open"=w202:bool)
            n90 = case shown="True" w202 {
              tunnel: [w208 w211] -> w207
              tunnel: w205 -> [w208 w210]
              tunnel: w203 -> [_ w209]
              frame False {
              }
              frame True {
                n91 = invoke class="VI" method="FP.Close"(reference=w209, error in=w210) -> (error out=w211:errorcluster)  [unwired: 1 in, 2 out]
              }
            }
          }
        }
        n92 = call <vilib>:"Add State(s) to Queue__jki_lib_state_machine.vi"("State(s) in (\"\")"=w189) -> ("States Out"=w188:string)  [unwired: 14 in]
      }
      frame "---------- Macro ----------" {
        # "Do not put any code in this frame.\n(It is a separator no-op. You can make a copy of this frame to create a new Macro frame)"
        n93 = call <vilib>:"Add State(s) to Queue__jki_lib_state_machine.vi"("State(s) in (\"\")"=w215) -> ("States Out"=w214:string)  [unwired: 14 in]
      }
      frame "Macro: Initialize" {
        w216 = "Data: Initialize\nInitialize Core Data\nUI: Initialize\nUI: Front Panel State >> Open"  # Data: Initialize Initialize Core Data UI: Initialize UI: Front Panel State >> Open
        # "Initialization Macro\n(This is called once, when the VI starts)"
        n94 = call <vilib>:"Add State(s) to Queue__jki_lib_state_machine.vi"("State(s) in Front (\"\")"=w216, "State(s) in (\"\")"=w220) -> ("States Out"=w219:string)  [unwired: 13 in]
      }
      frame "Macro: Exit" {
        # "Exit Macro\n(This is called once, when the VI exits)"
        n95 = Unbundle By Name(w227) -> ("Core.Close Panel on Exit?"=w226:bool)
        n96 = Select(t="UI: Front Panel State >> Close", s=w226, f="") -> (s? t:f=w223:string)
        n97 = call <vilib>:"Add State(s) to Queue__jki_lib_state_machine.vi"("State(s) in (\"\")"=w223, "State(s) at Back (\"\")"="Data: Cleanup\nExit") -> ("States Out"=w221:string)  [unwired: 13 in]
        n98 = call <vilib>:"Add State(s) to Queue__jki_lib_state_machine.vi"("State(s) in Front (\"\")"=w221, "State(s) in (\"\")"=w230) -> ("States Out"=w229:string)  [unwired: 13 in]
      }
      frame "---------- New Category ----------" {
        # "Template Separator\n(You can make a copy of, or modify, this frame)"
        n99 = call <vilib>:"Add State(s) to Queue__jki_lib_state_machine.vi"("State(s) in (\"\")"=w234) -> ("States Out"=w233:string)  [unwired: 14 in]
      }
      frame "Read ConcPressTemp" {
        # "Creates a rotating array for calculation of moving average"
        # "Calculates Mean, std, std error and std error precentages\nand output that results to graph and indicators"
        n100 = call "DAQ Assistant2"() -> ("data"=w241:dynamicdata)  [unwired: 17 in, 2 out]
        n101 = Unbundle(w291) -> (w290:dbl[], "Running Average Time(sec)"=w285:i32, "dup CPC port"=w238:refnum<visa-resource-name>, "CPC model"=w237:string, w273:cluster{dbl[], dbl[], "element":dbl}, w272:cluster{dbl[], dbl[], "element":dbl})  [unwired: 8 out]
        n102 = call "DAQ Assistant"() -> ("data"=w242:dynamicdata)  [unwired: 17 in, 2 out]
        n103 = case shown="False" "Allow SMPS scan" {
          tunnel: w238 -> [w298 _]
          tunnel: w237 -> [w297 _]
          tunnel: [w296 0.0 ("concentration part/cm3")] -> w235
          frame False {
            n104 = call "CPCReadlior.vi"("model"=w297, "CPC port"=w298) -> ("concentration part/cm3"=w296:dbl)  [unwired: 8 in, 1 out]
          }
          frame True {
          }
        }
        "Conc. (N/cm^3)" <- w235
        "CPCconc" <- w235
        n105 = call "Convert from Dynamic Data2"("Dynamic Data Type"=w241) -> ("Scalar"=w240:dbl)  [unwired: 3 in]
        "Pressure (Hectopascal)" <- w240
        n106 = Unbundle(w273) -> (w270:dbl[], w263:dbl[])  [unwired: 1 out]
        n107 = Unbundle(w272) -> (w268:dbl[], w261:dbl[])  [unwired: 1 out]
        n108 = Rotate 1D Array(1:w290, 2:1 ("n")) -> (0:w288:dbl[])
        n109 = Rotate 1D Array(1:w270, 2:1 ("n")) -> (0:w267:dbl[])
        n110 = Rotate 1D Array(1:w268, 2:1 ("n")) -> (0:w265:dbl[])
        n111 = call "Convert from Dynamic Data"("Dynamic Data Type"=w242) -> ("Scalar"=w239:dbl)  [unwired: 3 in]
        "Temperature(Celcius)" <- w239
        n112 = Replace Array Subset(array=w288, new element=w235, index=0.0 ("new element/subarray")) -> (w279:dbl[])
        "output array" <- w279
        n113 = Less?(x=w285, y=0) -> (x < y?=w243:bool)
        n114 = case shown="True" w243 {
          tunnel: [w330 w340] -> w283
          tunnel: w235 -> [w329 w341]
          tunnel: w279 -> [_ w336]
          tunnel: [w328 w338] -> w278
          tunnel: [w328 w337] -> w276
          tunnel: [w328 w333] -> w282
          tunnel: [w328 w331] -> w277
          frame False {
            w328 = 0 ("y")
            n115 = Bundle("concentration part/cm3"=w329, "concentration part/cm3"=w329) -> (w330:T6)  [unwired: 1 in]
          }
          frame True {
            n116 = Array Size(array=w336) -> (size(s)=w335:i32)
            n117 = Square Root(x=w335) -> (sqrt(x)=w334:dbl)
            n118 = call <vilib>:"Std Deviation and Variance.vi"("X"=w336) -> ("mean"=w337:dbl, "standard deviation"=w333:dbl)  [unwired: 1 in, 1 out]
            n119 = Divide(x=w333, y=w334) -> (x/y=w331:dbl)
            n120 = Divide(x=w331, y=w337) -> (x/y=w332:dbl)
            n121 = Multiply(x=w332, y=100.0) -> (x*y=w338:dbl)
            n122 = Bundle("concentration part/cm3"=w341, "mean"=w337) -> (w340:T7)  [unwired: 1 in]
          }
        }
        "Particle Concentration from CPC" <- w283
        "Std Error Conc. (%)" <- w278
        "Mean Conc." <- w276
        "Std Concentration" <- w282
        "Std Error Concentration" <- w277
        n123 = Replace Array Subset(array=w267, new element=w240, index=0) -> (w259:dbl[])
        n124 = Replace Array Subset(array=w265, new element=w239, index=0) -> (w258:dbl[])
        n125 = case shown="True" w243 {
          tunnel: [w316 w326] -> w256
          tunnel: w240 -> [w315 w327]
          tunnel: w259 -> [_ w322]
          tunnel: [w314 w324] -> w250
          tunnel: [w314 w323] -> w255
          tunnel: [w314 w319] -> _
          tunnel: [w314 w317] -> _
          frame False {
            w314 = 0 ("y")
            n126 = Bundle("Scalar"=w315, "Scalar"=w315) -> (w316:cluster{"Scalar":dbl, "Scalar":dbl})  [unwired: 1 in]
          }
          frame True {
            n127 = Array Size(array=w322) -> (size(s)=w321:i32)
            n128 = call <vilib>:"Std Deviation and Variance.vi"("X"=w322) -> ("mean"=w323:dbl, "standard deviation"=w319:dbl)  [unwired: 1 in, 1 out]
            n129 = Square Root(x=w321) -> (sqrt(x)=w320:dbl)
            n130 = Divide(x=w319, y=w320) -> (x/y=w317:dbl)
            n131 = Divide(x=w317, y=w323) -> (x/y=w318:dbl)
            n132 = Bundle("Scalar"=w327, "mean"=w323) -> (w326:cluster{"Scalar":dbl, "mean":dbl})  [unwired: 1 in]
            n133 = Multiply(x=w318, y=100.0) -> (x*y=w324:dbl)
          }
        }
        "Pressure Graph" <- w256
        "Mean Pressure" <- w255
        "Std Error Pressure (%)" <- w250
        n134 = case shown="True" w243 {
          tunnel: [w302 w312] -> w257
          tunnel: w239 -> [w301 w313]
          tunnel: w258 -> [_ w308]
          tunnel: [w300 w310] -> w245
          tunnel: [w300 w309] -> w254
          tunnel: [w300 w305] -> _
          tunnel: [w300 w303] -> _
          frame False {
            w300 = 0 ("y")
            n135 = Bundle("Scalar"=w301, "Scalar"=w301) -> (w302:cluster{"Scalar":dbl, "Scalar":dbl})  [unwired: 1 in]
          }
          frame True {
            n136 = Array Size(array=w308) -> (size(s)=w307:i32)
            n137 = Square Root(x=w307) -> (sqrt(x)=w306:dbl)
            n138 = call <vilib>:"Std Deviation and Variance.vi"("X"=w308) -> ("mean"=w309:dbl, "standard deviation"=w305:dbl)  [unwired: 1 in, 1 out]
            n139 = Divide(x=w305, y=w306) -> (x/y=w303:dbl)
            n140 = Divide(x=w303, y=w309) -> (x/y=w304:dbl)
            n141 = Bundle("Scalar"=w313, "mean"=w309) -> (w312:cluster{"Scalar":dbl, "mean":dbl})  [unwired: 1 in]
            n142 = Multiply(x=w304, y=100.0) -> (x*y=w310:dbl)
          }
        }
        "Temperature Graph" <- w257
        "Std Error Temp (%)" <- w245
        "Mean Temperature" <- w254
        n143 = Decrement(x=w285) -> (x-1=w286:i32)
        n144 = Bundle(w259, w263, "Scalar"=w240) -> (w262:cluster{dbl[], dbl[], "Scalar":dbl})  [unwired: 1 in]
        n145 = Bundle(w258, w261, "Scalar"=w239) -> (w260:cluster{dbl[], dbl[], "Scalar":dbl})  [unwired: 1 in]
        n146 = Bundle(cluster=w291, w279, "Running Average Time(sec)"=w286, "element"=w235, w262, w260) -> (w292:T3)  [unwired: 9 in]
        n147 = Greater?(x="Std Press. error tolerance(%)", y=w250) -> (0:w253:bool)
        n148 = Greater?(x="Std Temp error tolerance(%)", y=w245) -> (0:w248:bool)
        n149 = And(x=w253, y=w243) -> (x .and. y?=w252:bool)
        n150 = And(x=w248, y=w243) -> (x .and. y?=w247:bool)
        n151 = Greater?(x="Std Conc. error tolerance(%)", y=w278) -> (0:w280:bool)
        n152 = Not(x=w252) -> (.not. x?=w249:bool)
        n153 = Not(x=w247) -> (.not. x?=w244:bool)
        n154 = property on="Mean Pressure" class="DigNum (strict)"("Blinking"=w249) -> ()  [unwired: 2 in, 2 out]
        n155 = property on="Mean Temperature" class="DigNum (strict)"("Blinking"=w244) -> ()  [unwired: 2 in, 2 out]
        n156 = And(x=w280, y=w243) -> (x .and. y?=w275:bool)
        n157 = Not(x=w275) -> (.not. x?=w274:bool)
        n158 = property on="Mean Conc." class="DigNum (strict)"("Blinking"=w274) -> ()  [unwired: 2 in, 2 out]
        n159 = call <vilib>:"Add State(s) to Queue__jki_lib_state_machine.vi"("State(s) in (\"\")"=w295) -> ("States Out"=w294:string)  [unwired: 14 in]
      }
      frame "New Category: 2" {
        # "Your code here.\n(You can make a copy of, or modify, this frame)"
        n160 = call <vilib>:"Add State(s) to Queue__jki_lib_state_machine.vi"("State(s) in (\"\")"=w345) -> ("States Out"=w344:string)  [unwired: 14 in]
      }
      frame "Take Measurement" {
        # "Incase andor script is aborted\ninitiate a timeout of 3 min in recording the data and reinitialize to zero"
        # "Your code here.\n(You can make a copy of, or modify, this frame)"
        n161 = Unbundle(w369) -> (w370:dbl[], "element"=w372:dbl, w357:cluster{dbl[], dbl[], "element":dbl}, w356:cluster{dbl[], dbl[], "element":dbl})  [unwired: 10 out]
        n162 = property on="Saving in Progress" class="Slide (strict)"("Caption.Visible"=TRUE) -> ()  [unwired: 2 in, 2 out]
        n163 = Unbundle(w357) -> (w351:dbl[], w355:dbl[], "element"=w352:dbl)
        n164 = Unbundle(w356) -> (w348:dbl[], w354:dbl[], "element"=w347:dbl)
        n165 = Insert Into Array(array=w370, index=0, new element=w372) -> (w367:dbl[])
        "output array 2" <- w367
        n166 = Insert Into Array(array=w355, index=0, new element=w352) -> (w353:dbl[])
        n167 = Insert Into Array(array=w354, index=0, new element=w347) -> (w349:dbl[])
        n168 = Array Size(array=w367) -> (size(s)=w363:i32)
        n169 = Bundle(w351, w353, "element"=w352) -> (w350:cluster{dbl[], dbl[], "element":dbl})  [unwired: 1 in]
        n170 = Bundle(w348, w349, "element"=w347) -> (w346:cluster{dbl[], dbl[], "element":dbl})  [unwired: 1 in]
        n171 = Quotient & Remainder(x=w363, y=10) -> (x-y*floor(x/y)=→"Saving in Progress":i32)  [unwired: 1 out]
        n172 = Greater?(x=w363, y=300) -> (0:w361:bool)
        n173 = Bundle(cluster=w369, w367, "dimension size"=w363, w350, w346) -> (w368:T3)  [unwired: 10 in]
        n174 = case shown="True" w361 {
          tunnel: ["" ("State(s) in Front (\"\")") "Write to file" ("State(s) in Front (\"\")")] -> w360
          frame False {
          }
          frame True {
          }
        }
        n175 = call <vilib>:"Add State(s) to Queue__jki_lib_state_machine.vi"("State(s) in Front (\"\")"=w360, "State(s) in (\"\")"=w375) -> ("States Out"=w374:string)  [unwired: 13 in]
      }
      frame "Write to file" {
        # "Initialize mean after it is written to file"
        n176 = Unbundle(w424) -> (w432:dbl[], "input file"=w415:path, "input file"=w416:path, "input file"=w402:path, "input file"=w401:path, w412:cluster{dbl[], dbl[], "element":dbl}, w411:cluster{dbl[], dbl[], "element":dbl})  [unwired: 7 out]
        n177 = property on="Saving in Progress" class="Slide (strict)"("Caption.Visible"=FALSE) -> ()  [unwired: 2 in, 2 out]
        n178 = property on="Saving in Progress" class="Slide (strict)"("Value"=0 ("Saving in Progress")) -> ()  [unwired: 2 in, 2 out]
        n179 = Array Size(array=w432) -> (size(s)=w429:i32)
        "Number Samples of Conc." <- w429
        n180 = Delete(path (use dialog)=w415, error in=w413) -> (deleted path=w414:path, error out=w399:errorcluster)  [unwired: 3 in, 1 out]
        n181 = Delete(path (use dialog)=w402, error in=w399) -> (deleted path=w394:path, error out=w400:errorcluster)  [unwired: 3 in, 1 out]
        n182 = Delete(path (use dialog)=w401, error in=w400) -> (deleted path=w390:path, error out=w398:errorcluster)  [unwired: 3 in, 1 out]
        n183 = call <vilib>:"Std Deviation and Variance.vi"("X"=w432) -> ("mean"=w427:dbl, "standard deviation"=w431:dbl)  [unwired: 1 in, 1 out]
        "Mean conc. to file (N/cm^3)" <- w427
        n184 = Unbundle(w412) -> (w389:dbl[], w410:dbl[], "element"=w388:dbl)
        n185 = Unbundle(w411) -> (w387:dbl[], w405:dbl[], "element"=w386:dbl)
        n186 = Format Into String(format string="%d %d", initial string=w416, 0.0 ("input 1"), 0.0 ("input 2")) -> ()  [unwired: 1 in, 2 out]
        n187 = Array Size(array=w410) -> (size(s)=w403:i32)
        "Number Samples of Press." <- w403
        n188 = call <vilib>:"Std Deviation and Variance.vi"("X"=w410) -> ("mean"=w396:dbl, "standard deviation"=w408:dbl)  [unwired: 1 in, 1 out]
        "Mean Press. to file (hpas)" <- w396
        n189 = Square Root(x=w429) -> (sqrt(x)=w433:dbl)
        n190 = Array Size(array=w405) -> (size(s)=w404:i32)
        "Number Samples of Temp" <- w404
        n191 = call <vilib>:"Std Deviation and Variance.vi"("X"=w405) -> ("mean"=w392:dbl, "standard deviation"=w406:dbl)  [unwired: 1 in, 1 out]
        "Mean Temp to file (deg)" <- w392
        n192 = Square Root(x=w403) -> (sqrt(x)=w409:dbl)
        n193 = Square Root(x=w404) -> (sqrt(x)=w407:dbl)
        n194 = Divide(x=w431, y=w433) -> (x/y=w428:dbl)
        "Std error to file (N/cm^3)" <- w428
        n195 = Divide(x=w408, y=w409) -> (x/y=w395:dbl)
        "Std error Press. to file (hpas)" <- w395
        n196 = Divide(x=w406, y=w407) -> (x/y=w391:dbl)
        "Std error Temp to file (deg)" <- w391
        n197 = Format Into String(format string="%f, %f,", initial string=w414, w427, w428) -> ()  [unwired: 1 in, 2 out]
        n198 = Format Into String(format string="%f, %f,", initial string=w394, w396, w395) -> ()  [unwired: 1 in, 2 out]
        n199 = Format Into String(format string="%f, %f,", initial string=w390, w392, w391) -> ()  [unwired: 1 in, 2 out]
        n200 = Initialize Array(0.0 ("element"), 0 ("dimension size")) -> (w383:dbl[])
        n201 = Initialize Array(0.0 ("element"), 0 ("dimension size")) -> (w380:dbl[])
        n202 = Bundle(w387, w383, "element"=w386) -> (w378:cluster{dbl[], dbl[], "element":dbl})  [unwired: 1 in]
        n203 = Bundle(w389, w380, "element"=w388) -> (w379:cluster{dbl[], dbl[], "element":dbl})  [unwired: 1 in]
        n204 = Initialize Array(0.0 ("element"), 0 ("dimension size")) -> (w422:dbl[])
        n205 = Bundle(cluster=w424, w422, w379, w378) -> (w423:T3)  [unwired: 11 in]
        n206 = call <vilib>:"Add State(s) to Queue__jki_lib_state_machine.vi"("State(s) in (\"\")"=w435) -> ("States Out"=w434:string)  [unwired: 14 in]
      }
    }
  }
